vi "6133_SaveToTDMS.vi"(11 "数据":T1={"时间"=timestamp(3515985789.500352 s since 1904-01-01), "声发射"=array[32000 elements], "电涡流1"=array[32000 elements], "电涡流2"=array[32000 elements], "电涡流3"=array[32000 elements], "电涡流4"=array[32000 elements], "电涡流5"=array[32000 elements], "加速度1"=array[80000 elements], "加速度2"=array[80000 elements]}) -> (3 "错误输出":errorcluster)   [LabVIEW 2014]
panel:
  in  "文件名":string="6133"
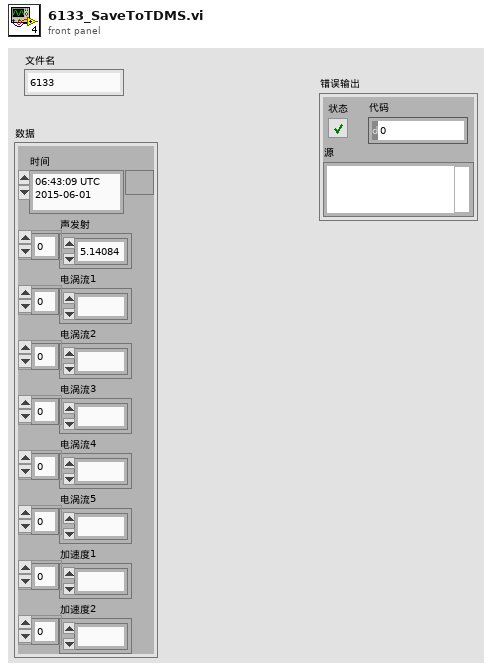
[diagram p1: front panel]
types:
  T1 = cluster{"时间":timestamp, "声发射":sgl[], "电涡流1":sgl[], "电涡流2":sgl[], "电涡流3":sgl[], "电涡流4":sgl[], "电涡流5":sgl[], "加速度1":sgl[], "加速度2":sgl[]}
  T2 = enum16{"open", "open or create", "create or replace", "create", "open (read-only)"}
  T3 = cluster{"字符串":string, "字符串 2":string, "字符串 3":string, "字符串 4":string, "字符串 5":string, "字符串 6":string, "字符串 7":string, "字符串 8":string}
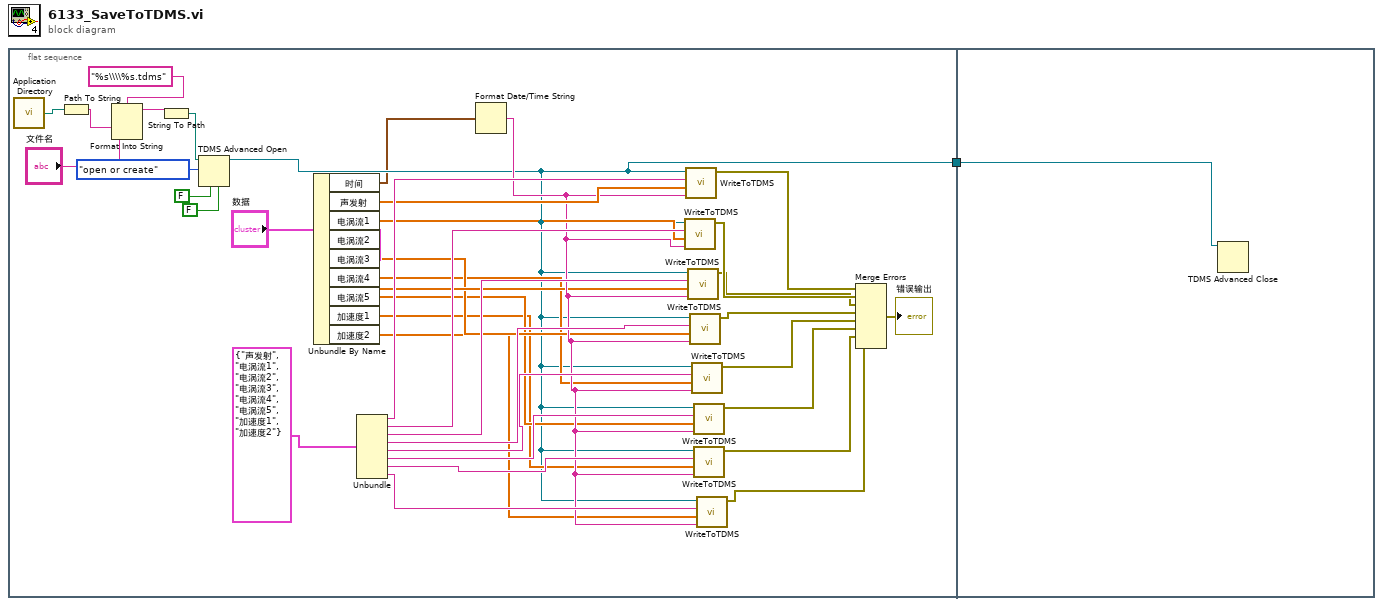
[diagram p0: block diagram]
diagram:
  n1 = flat-sequence {
    tunnel: [w5] -> w1
    tunnel: w1 -> [w41]
    frame #0 {
      n2 = call <vilib>:"Application Directory.vi"() -> ("Application Directory"=w38:path)
      n3 = Path To String(path=w38) -> (string=w39:string)
      n4 = Format Into String(format string="%s\\\\%s.tdms", w39, "文件名") -> (resulting string=w40:string)  [unwired: 2 in, 1 out]
      n5 = String To Path(string=w40) -> (path=w36:path)
      n6 = TDMS Advanced Open(4:FALSE ("启用异步？(T)"), 6:FALSE ("禁用缓冲？(T)"), 10:T2."open or create" ("操作(0:open)"), 11:w36) -> (3:w5:refnum<k34>)  [unwired: 1 in, 2 out]
      n7 = Unbundle By Name("数据") -> ("时间"=w3:timestamp, "声发射"=w30:sgl[], "电涡流1"=w22:sgl[], "电涡流2"=w20:sgl[], "电涡流3"=w19:sgl[], "电涡流4"=w18:sgl[], "电涡流5"=w17:sgl[], "加速度1"=w16:sgl[], "加速度2"=w15:sgl[])
      n8 = Unbundle(T3 {"字符串"="声发射", "字符串 2"="电涡流1", "字符串 3"="电涡流2", "字符串 4"="电涡流3", "字符串 5"="电涡流4", "字符串 6"="电涡流5", "字符串 7"="加速度1", "字符串 8"="加速度2"} ("簇")) -> ("字符串"=w31:string, "字符串 2"=w29:string, "字符串 3"=w28:string, "字符串 4"=w27:string, "字符串 5"=w26:string, "字符串 6"=w25:string, "字符串 7"=w24:string, "字符串 8"=w23:string)
      n9 = Format Date/Time String(seconds (now)=w3) -> (date/time string=w21:string)  [unwired: 2 in]
      n10 = call "WriteToTDMS.vi"("组名称（未命名）"=w21, "数据"=w22, "通道名"=w29, "tdms文件"=w5) -> ("错误输出"=w13:errorcluster)  [unwired: 7 in]
      n11 = call "WriteToTDMS.vi"("组名称（未命名）"=w21, "数据"=w30, "通道名"=w31, "tdms文件"=w5) -> ("错误输出"=w14:errorcluster)  [unwired: 7 in]
      n12 = call "WriteToTDMS.vi"("组名称（未命名）"=w21, "数据"=w20, "通道名"=w28, "tdms文件"=w5) -> ("错误输出"=w12:errorcluster)  [unwired: 7 in]
      n13 = call "WriteToTDMS.vi"("组名称（未命名）"=w21, "数据"=w19, "通道名"=w27, "tdms文件"=w5) -> ("错误输出"=w11:errorcluster)  [unwired: 7 in]
      n14 = call "WriteToTDMS.vi"("组名称（未命名）"=w21, "数据"=w18, "通道名"=w26, "tdms文件"=w5) -> ("错误输出"=w10:errorcluster)  [unwired: 7 in]
      n15 = call "WriteToTDMS.vi"("组名称（未命名）"=w21, "数据"=w17, "通道名"=w25, "tdms文件"=w5) -> ("错误输出"=w9:errorcluster)  [unwired: 7 in]
      n16 = call "WriteToTDMS.vi"("组名称（未命名）"=w21, "数据"=w16, "通道名"=w24, "tdms文件"=w5) -> ("错误输出"=w8:errorcluster)  [unwired: 7 in]
      n17 = call "WriteToTDMS.vi"("组名称（未命名）"=w21, "数据"=w15, "通道名"=w23, "tdms文件"=w5) -> ("错误输出"=w7:errorcluster)  [unwired: 7 in]
      n18 = Merge Errors(w14, w13, w12, w11, w10, w9, w8, w7) -> (→"错误输出":errorcluster)
    }
    frame #1 {
      n19 = TDMS Advanced Close(11:w41) -> ()  [unwired: 3 in, 2 out]
    }
  }
